vi "Write File Path Control.vi"(8 "error in (no error)":errorcluster, 10 "Measurement Locations":path[](array[path]), 11 "Load Measurements Message in":refnum<class "Find Measurements On Disk Message.lvclass">) -> (0 "error out":errorcluster, 3 "Load Measurements Message out":refnum<class "Find Measurements On Disk Message.lvclass">)   [LabVIEW 2015, in "Controller Actor.lvlib" / "Find Measurements On Disk Message.lvclass"]
uses:
  Find Measurements On Disk Message.lvclass
  Find Measurements On Disk Message.lvclass/Find Measurements On Disk Message.ctl
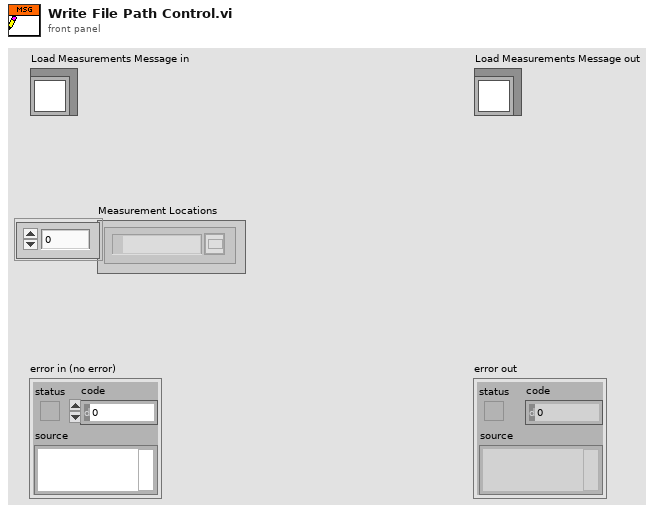
[diagram p1: front panel]
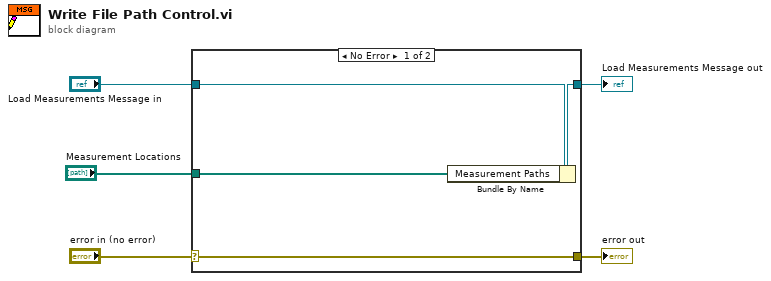
[diagram p0: block diagram]
diagram:
  n1 = case shown="No Error" "error in (no error)" {
    selector: "error in (no error)" -> [w9 w10]
    tunnel: [w9 w10] -> w4
    tunnel: [w7 w11] -> w2
    tunnel: "Load Measurements Message in" -> [w8 w11]
    tunnel: "Measurement Locations" -> [w6 _]
    frame No Error {
      n2 = Bundle By Name(cluster=w8, "Measurement Paths"=w6) -> (w7:refnum<class "Find Measurements On Disk Message.lvclass">)
    }
    frame Error {
    }
  }
  "error out" <- w4
  "Load Measurements Message out" <- w2
